vi "SerialLogic.vi"(8 "read buffer":string, 11 "COM PORT":refnum<visa-resource-name>) -> (3 "RX_DATA":i32[](array[numeric]))   [LabVIEW 2021]
uses:
  <vilib>/Instr/_visa.llb/VISA Configure Serial Port (Instr).vi
panel:
  out "Calc_Check":i32
  out "rx_CheckSum":i32
  out "number 10":i32
  out "number 9":i32
  out "number 8":i32
  out "number 7":i32
  out "number 6":i32
  out "number 5":i32
  out "number 4":i32
  out "number 3":i32
  out "LENGHT":i32
  out "ID":i32
  out "error in (no error)":errorcluster
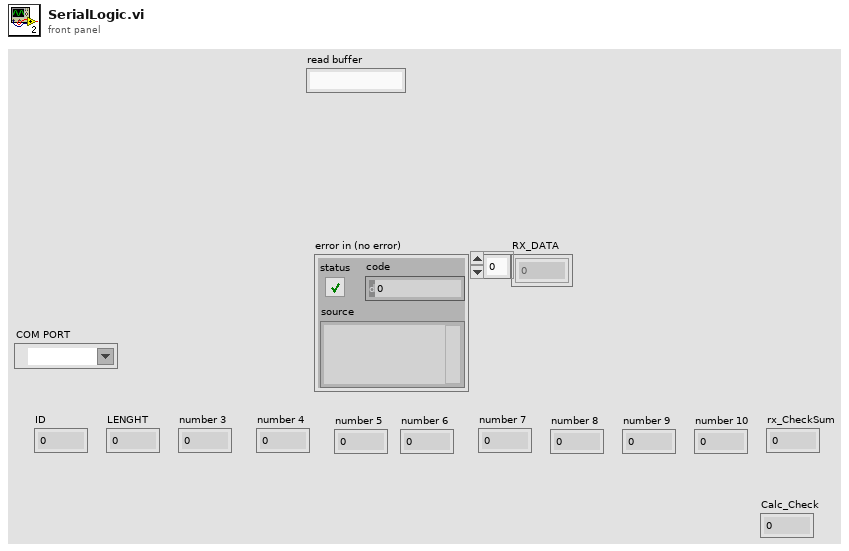
[diagram p1: front panel]
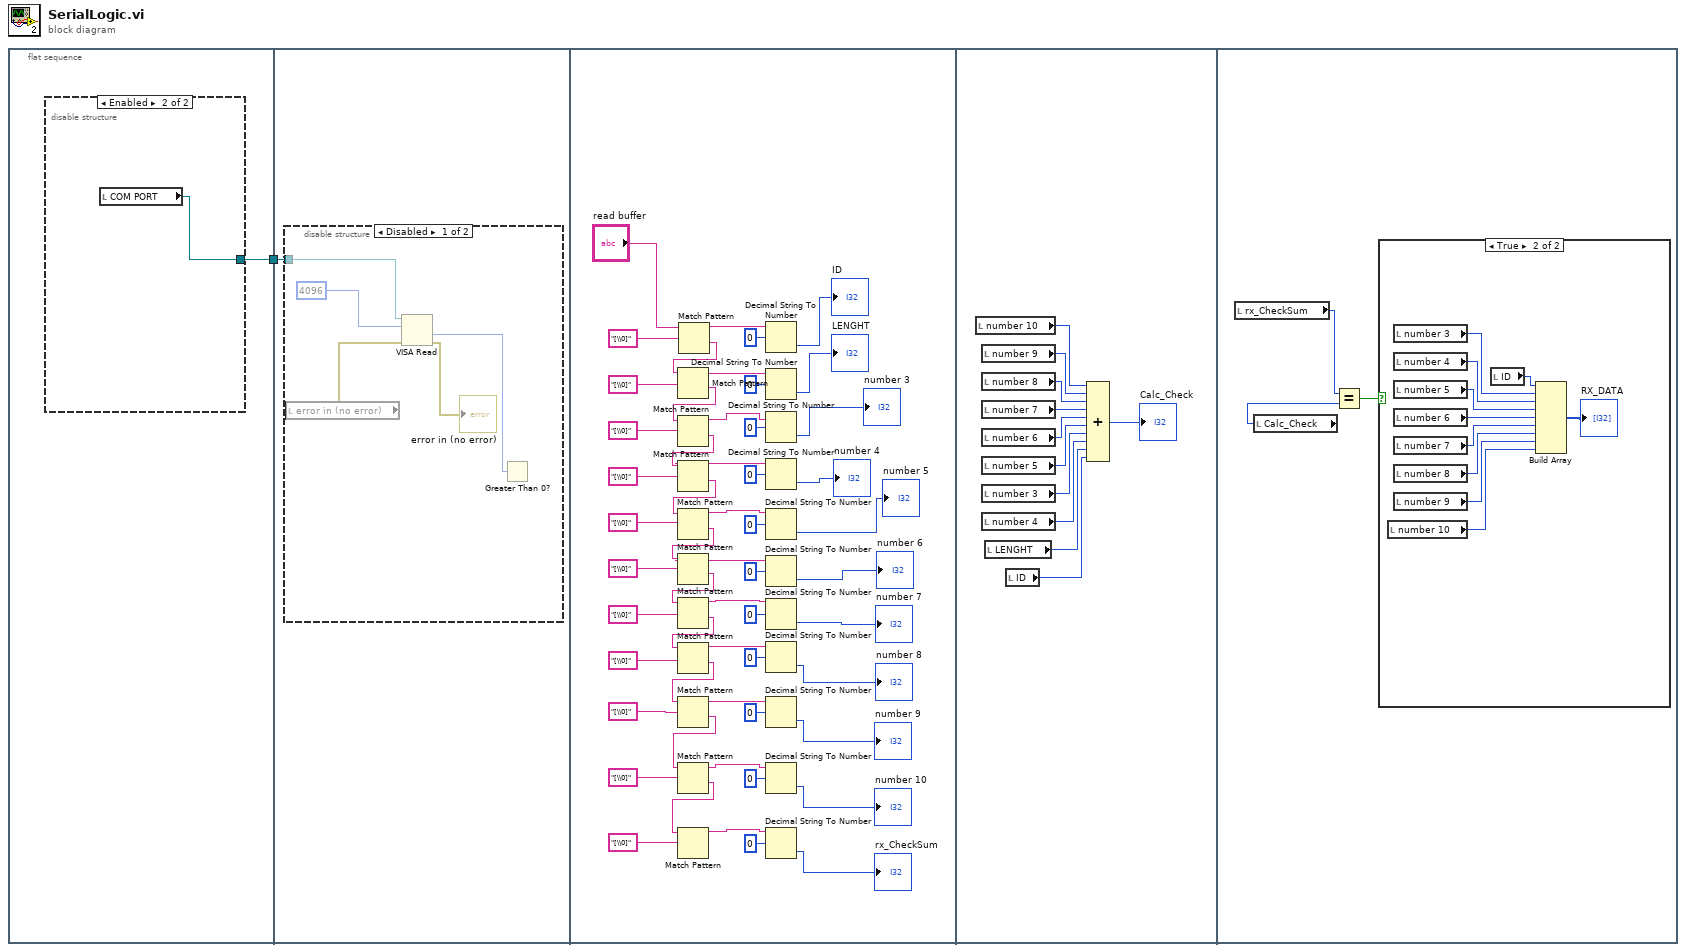
[diagram p0: block diagram]
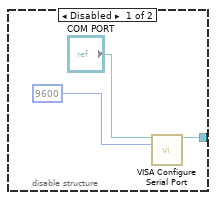
[diagram p2: hidden frame]
diagram:
  n1 = flat-sequence {
    tunnel: [w2] -> w1
    tunnel: w1 -> [w7]
    frame #0 {
      n2 = disable-structure shown="Enabled" {
        disable-tunnel: [w4 w6] -> w2
        frame Disabled {
          n3 = call-poly "VISA Configure Serial Port"("VISA resource name"="COM PORT", "baud rate (9600)"=u32 9600) -> ("VISA resource name out"=w4:refnum<visa-resource-name>)  [unwired: 12 in, 1 out]
        }
        frame Enabled {
          n4 = local read "COM PORT"() -> (w6:refnum<visa-resource-name>)
        }
      }
    }
    frame #1 {
      n5 = disable-structure shown="Disabled" {
        disable-tunnel: w7 -> [w13 _]
        frame Disabled {
          n6 = local read "error in (no error)"() -> (w10:errorcluster)
          n7 = VISA Read(VISA resource name=w13, byte count=u32 4096, error in (no error)=w10) -> (return count=w9:u32, error out=→"error in (no error)":errorcluster)  [unwired: 2 out]
          n8 = Greater Than 0?(x=w9) -> (x > 0?=w8:bool)
        }
        frame Enabled {
        }
      }
    }
    frame #2 {
      n9 = Match Pattern(string="read buffer", regular expression="[\\0]") -> (before substring=w59:string, after substring=w67:string)  [unwired: 1 in, 2 out]
      n10 = Match Pattern(string=w67, regular expression="[\\0]") -> (before substring=w58:string, after substring=w66:string)  [unwired: 1 in, 2 out]
      n11 = Match Pattern(string=w66, regular expression="[\\0]") -> (before substring=w57:string, after substring=w65:string)  [unwired: 1 in, 2 out]
      n12 = Match Pattern(string=w65, regular expression="[\\0]") -> (before substring=w56:string, after substring=w64:string)  [unwired: 1 in, 2 out]
      n13 = Match Pattern(string=w64, regular expression="[\\0]") -> (before substring=w55:string, after substring=w63:string)  [unwired: 1 in, 2 out]
      n14 = Match Pattern(string=w63, regular expression="[\\0]") -> (before substring=w54:string, after substring=w62:string)  [unwired: 1 in, 2 out]
      n15 = Match Pattern(string=w62, regular expression="[\\0]") -> (before substring=w53:string, after substring=w61:string)  [unwired: 1 in, 2 out]
      n16 = Match Pattern(string=w61, regular expression="[\\0]") -> (before substring=w52:string, after substring=w60:string)  [unwired: 1 in, 2 out]
      n17 = Match Pattern(string=w60, regular expression="[\\0]") -> (before substring=w51:string, after substring=w24:string)  [unwired: 1 in, 2 out]
      n18 = Match Pattern(string=w24, regular expression="[\\0]") -> (before substring=w21:string, after substring=w18:string)  [unwired: 1 in, 2 out]
      n19 = Match Pattern(string=w18, regular expression="[\\0]") -> (before substring=w17:string)  [unwired: 1 in, 3 out]
      n20 = Decimal String To Number(string=w59, offset=0) -> (number=→"ID":i32)  [unwired: 1 in, 1 out]
      n21 = Decimal String To Number(string=w58, offset=0) -> (number=→"LENGHT":i32)  [unwired: 1 in, 1 out]
      n22 = Decimal String To Number(string=w57, offset=0) -> (number=→"number 3":i32)  [unwired: 1 in, 1 out]
      n23 = Decimal String To Number(string=w56, offset=0) -> (number=→"number 4":i32)  [unwired: 1 in, 1 out]
      n24 = Decimal String To Number(string=w55, offset=0) -> (number=→"number 5":i32)  [unwired: 1 in, 1 out]
      n25 = Decimal String To Number(string=w54, offset=0) -> (number=→"number 6":i32)  [unwired: 1 in, 1 out]
      n26 = Decimal String To Number(string=w53, offset=0) -> (number=→"number 7":i32)  [unwired: 1 in, 1 out]
      n27 = Decimal String To Number(string=w52, offset=0) -> (number=→"number 8":i32)  [unwired: 1 in, 1 out]
      n28 = Decimal String To Number(string=w51, offset=0) -> (number=→"number 9":i32)  [unwired: 1 in, 1 out]
      n29 = Decimal String To Number(string=w21, offset=0) -> (number=→"number 10":i32)  [unwired: 1 in, 1 out]
      n30 = Decimal String To Number(string=w17, offset=0) -> (number=→"rx_CheckSum":i32)  [unwired: 1 in, 1 out]
    }
    frame #3 {
      n31 = local read "number 10"() -> (w70:i32)
      n32 = local read "number 9"() -> (w71:i32)
      n33 = local read "number 8"() -> (w72:i32)
      n34 = local read "number 7"() -> (w73:i32)
      n35 = local read "number 6"() -> (w74:i32)
      n36 = local read "number 5"() -> (w75:i32)
      n37 = local read "number 3"() -> (w76:i32)
      n38 = local read "number 4"() -> (w77:i32)
      n39 = local read "LENGHT"() -> (w78:i32)
      n40 = local read "ID"() -> (w79:i32)
      n41 = Compound Arithmetic op=ADD(w70, w71, w72, w73, w74, w75, w76, w77, w78, w79) -> (→"Calc_Check":i32)
    }
    frame #4 {
      n42 = local read "rx_CheckSum"() -> (w82:i32)
      n43 = local read "Calc_Check"() -> (w81:i32)
      n44 = Equal?(x=w82, y=w81) -> (x = y?=w80:bool)
      n45 = case shown="True" w80 {
        frame False {
        }
        frame True {
          n46 = local read "number 10"() -> (w84:i32)
          n47 = local read "number 3"() -> (w91:i32)
          n48 = local read "number 4"() -> (w90:i32)
          n49 = local read "number 5"() -> (w89:i32)
          n50 = local read "number 6"() -> (w88:i32)
          n51 = local read "number 7"() -> (w87:i32)
          n52 = local read "number 8"() -> (w86:i32)
          n53 = local read "number 9"() -> (w85:i32)
          n54 = local read "ID"() -> (w92:i32)
          n55 = Build Array(w92, w91, w90, w89, w88, w87, w86, w85, w84) -> (→"RX_DATA":i32[])
        }
      }
    }
  }
